vi "趋势图对话框.vi"(9 "参数":string, 10 "Array输入":refnum<vi>, 11 "原点":T1 caption="点") -> ()   [LabVIEW 2016, in "多参数状态显示.xctl"]
uses:
  <vilib>/Utility/miscctls.llb/LVPointTypeDef.ctl
panel:
  out "波形图":dbl[](graph)
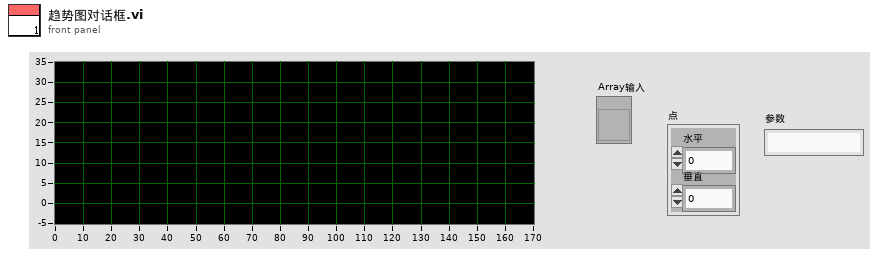
[diagram p1: front panel]
types:
  T1 = typedef "LVPointTypeDef.ctl" = cluster{"Horizontal":i16, "Vertical":i16}
  T2 = typedef "LVRectTypeDef.ctl" = cluster{"Left":i16, "Top":i16, "Right":i16, "Bottom":i16}
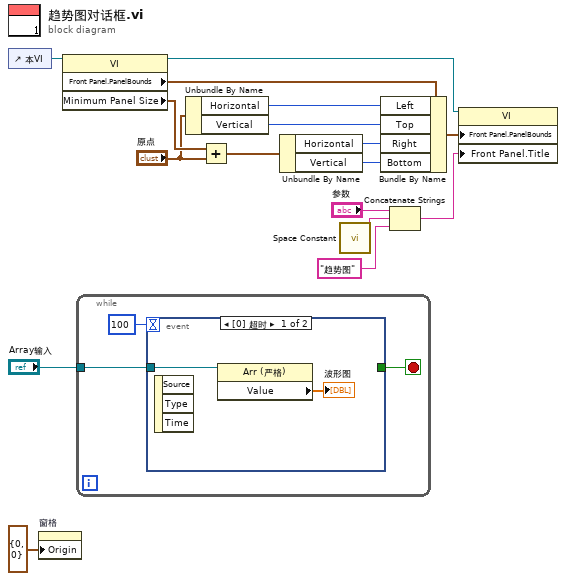
[diagram p0: block diagram]
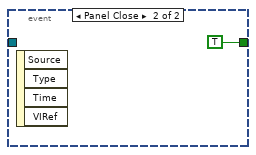
[diagram p2: hidden frame]
diagram:
  n1 = control-ref of="本VI"() -> (w16:refnum<vi>)
  n2 = property on="窗格" class="Pane"("Origin"=T1 {"Horizontal"=0, "Vertical"=0} ("原点")) -> ()  [unwired: 2 in, 2 out]
  n3 = property class="VI"(reference=w16) -> (reference out=w15:refnum<vi>, "Front Panel.PanelBounds"=w14:T2, "Minimum Panel Size"=w10:T1)  [unwired: 1 in, 1 out]
  n4 = while {
    tunnel: "Array输入" -> [w18]
    stop <- w20 stop-if-true
    n5 = event shown="[0] 超时" {
      selector: _ -> [_ _]
      dyn-events: _ -> [_ _]
      timeout: 100 -> [_ _]
      tunnel: [_ TRUE] -> w20
      tunnel: w18 -> [w22 _]
      event Timeout {
        n6 = event-data() -> ()  [unwired: 1 in, 3 out]
        n7 = property class="Arr (严格)"(reference=w22) -> ("Value"=→"波形图":dbl[])  [unwired: 1 in, 2 out]
      }
      event Panel Close {
        n8 = event-data() -> ()  [unwired: 1 in, 4 out]
      }
    }
  }
  n9 = Unbundle By Name("原点") -> ("Horizontal"=w12:i16, "Vertical"=w11:i16)
  n10 = Add(x=w10, y="原点") -> (x+y=w8:T1)
  n11 = Unbundle By Name(w8) -> ("Horizontal"=w7:i16, "Vertical"=w6:i16)
  n12 = call <vilib>:"Space Constant.vi"() -> ("String"=w1:string)
  n13 = Bundle By Name(cluster=w14, "Left"=w12, "Top"=w11, "Right"=w7, "Bottom"=w6) -> (w13:T2)
  n14 = Concatenate Strings("参数", w1, "趋势图" ("字符串")) -> (w3:string)
  n15 = property class="VI"(reference=w15, "Front Panel.PanelBounds"=w13, "Front Panel.Title"=w3) -> ()  [unwired: 1 in, 2 out]
